vi "Channel In Range.vi"(9 "All Channels (T)":bool=TRUE, 10 "Channel Index":i32, 11 "Mixer in":refnum<class "Mixer.lvclass">) -> (0 "error out":errorcluster, 2 "In Range":bool, 3 "Mixer out":refnum<class "Mixer.lvclass">)   [LabVIEW 2020, in "G-Audio.lvlib" / "Mixer.lvclass"]
uses:
  Mixer.lvclass
  Mixer.lvclass/Mixer.ctl
  <vilib>/Utility/error.llb/Error Cluster From Error Code.vi
  <vilib>/ErrorRing/Error Ring.xnode
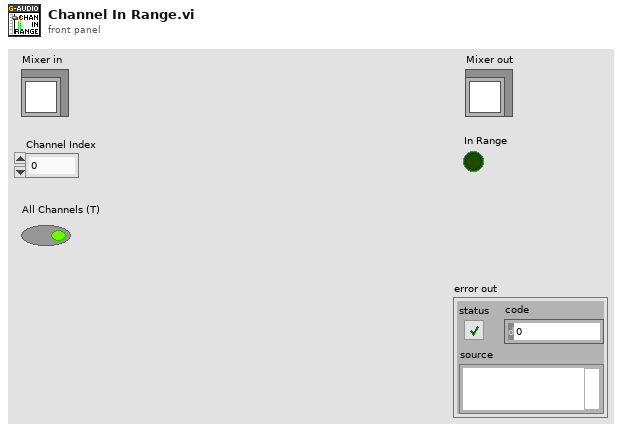
[diagram p1: front panel]
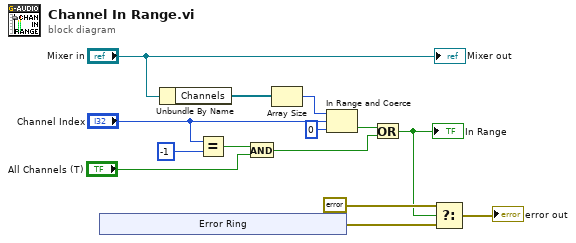
[diagram p0: block diagram]
diagram:
  n1 = xnode "Error Ring"() -> ("error out"=w10:errorcluster)
  n2 = Unbundle By Name("Mixer in") -> ("Channels"=w13:refnum<data-value>[])
  n3 = Equal?(x="Channel Index", y=-1) -> (x = y?=w5:bool)
  n4 = And(x=w5, y="All Channels (T)") -> (x .and. y?=w2:bool)
  n5 = Array Size(array=w13) -> (size(s)=w12:i32)
  n6 = In Range and Coerce(upper limit=w12, x="Channel Index", lower limit=0) -> (In Range?=w11:bool)  [unwired: 1 out]
  n7 = Or(x=w11, y=w2) -> (x .or. y?=w3:bool)
  "In Range" <- w3
  n8 = Select(t=errorcluster {"status"=FALSE, "code"=0, "source"=""}, s=w3, f=w10) -> (s? t:f=→"error out":errorcluster)
  "Mixer out" <- "Mixer in"
